vi "NavigateTryingToKeepPath.vi"(1 "Move Type":T1(ring)) -> ()   [LabVIEW 2015, in "Navigation2017.lvlib"]
uses:
  Navigation2017.lvlib
  MovementControl2017.lvlib
  Vector.ctl
  Navigation2017-util.lvlib
  Navigation2017-SubVIs.lvlib
  PathfindingSettings.ctl
  MovementSettings.ctl
  PathCostWeights.ctl
  IntermediatePositionGrids.ctl
panel:
  in  "Reached Next Path Point Threshold Distance (m)":dbl(knob) scale=0.0..1.0
  in  "Time to move 1m (TODO: consider speed?)":u32
  in  "Robot Speed":dbl(slide) scale=0.0..1.0
  in  "Dead Reckoning Move Distance (m)":dbl(knob) scale=0.5..4.0
  in  "Turning Radius (m)":dbl(knob) scale=0.75..4.0
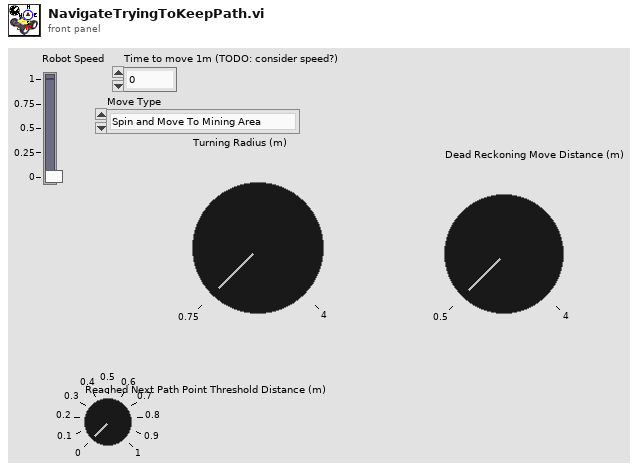
[diagram p1: front panel]
types:
  T1 = enum16{"Spin and Move To Mining Area", "Move To Collector Trough", "Move To Mining Area"}
  T2 = typedef "Navigation2017.lvlib/Vector.ctl" = cluster{"x":dbl, "y":dbl, "angle":dbl}
  T3 = typedef "LocalizationStatus.ctl" = cluster{"x":dbl, "y":dbl, "angle":dbl, "valid":bool, "lastUpdatedTime":dbl}
  T4 = typedef "Navigation2017.lvlib/PathfindingSettings.ctl" = cluster{"Movement Settings":T5, "Dead Zone":dbl, "Max Moves":dbl, "Move Segment Length (m)":dbl, "Path Cost Weights":T6, "Desperation - Reduction Per Attempt (Ratio)":dbl, "Desperation - Max Attempts":i16, "Log All Move Points":bool, "Intermediate Position Grids":T7}
  T5 = typedef "Navigation2017.lvlib/MovementSettings.ctl" = cluster{"Arrival Tolerance (m)":dbl, "Closeness Threshold (m)":dbl, "Pit Obstacle Radius (m)":dbl, "Pit Locations":cluster{"x":dbl, "y":dbl}[]}
  T6 = typedef "Navigation2017.lvlib/PathCostWeights.ctl" = cluster{"Length Weight":dbl, "Angle Weight":dbl, "Angle Error Weight":dbl, "Angle Error Threshold":dbl, "Per Move Penalty":dbl, "Closeness Weight":dbl, "Too Short Penalty":dbl, "Too Short Threshold":dbl}
  T7 = typedef "Navigation2017.lvlib/IntermediatePositionGrids.ctl" = cluster{"x1":dbl, "x2":dbl, "resolution":dbl}[]
  T8 = typedef "Navigation2017.lvlib/PathOfMoves.ctl" = cluster{"Dest Angle Error":dbl, "Dest Angle Considered":bool, "Moves":T9[]}
  T9 = typedef "Navigation2017.lvlib/Move.ctl" = cluster{"Did Reach Dest":bool, "Did Collide":bool, "Sum of Angle Changes (rad)":dbl, "Move Length (m)":dbl, "Closeness Sum":dbl, "Positions Along Move":cluster{"x":dbl, "y":dbl, "angle":dbl}[], "Moved Fwd":bool}
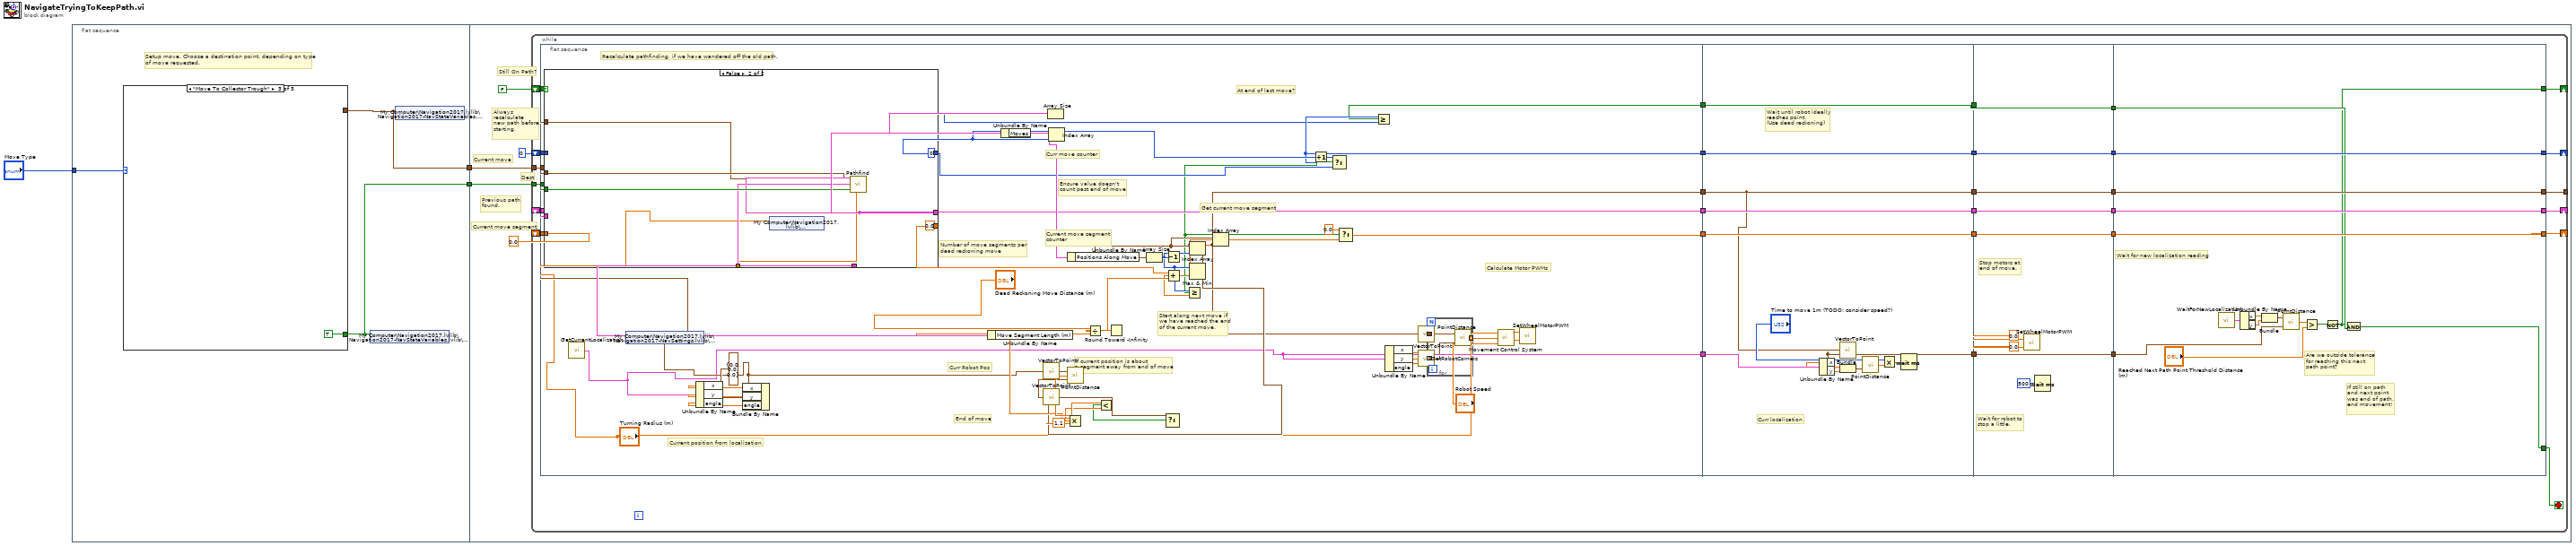
[diagram p0: block diagram]
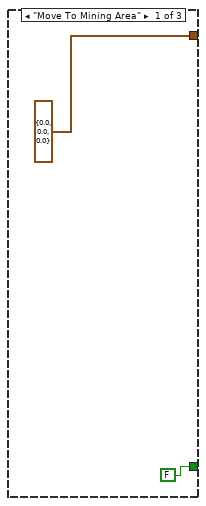
[diagram p2: hidden frame]
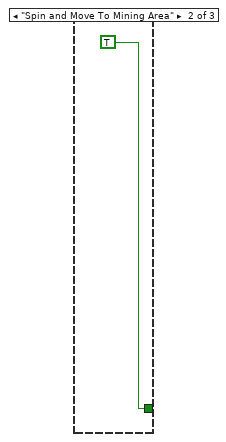
[diagram p3: hidden frame]
diagram:
  n1 = flat-sequence {
    tunnel: "Move Type" -> [w6]
    tunnel: [w5] -> w2
    tunnel: [w4] -> w1
    tunnel: w2 -> [w14]
    tunnel: w1 -> [w13]
    frame #0 {
      # "Setup move. Choose a destination point, depending on type\nof move requested."
      n2 = case shown="\"Move To Collector Trough\"" w6 {
        tunnel: [T2 {"x"=0.0, "y"=0.0, "angle"=0.0} ("Vector") _ _] -> w4
        tunnel: [FALSE TRUE TRUE] -> w5
        frame "Move To Mining Area" {
        }
        frame "Spin and Move To Mining Area" {
        }
        frame "Move To Collector Trough" {
        }
      }
      n3 = shared-variable "My Computer\\Navigation2017.lvlib\\Navigation2017-NavStateVariables.lvlib\\SpecifyingEndAngle"(w5) -> ()  [unwired: 1 in, 1 out]
      n4 = shared-variable "My Computer\\Navigation2017.lvlib\\Navigation2017-NavStateVariables.lvlib\\DestinationPoint"(w4) -> ()  [unwired: 1 in, 1 out]
    }
    frame #1 {
      # "Dest"
      # "Current move"
      # "Current move segment"
      # "Always \nrecalculate\nnew path before\nstarting."
      # "Previous path\nfound."
      # "Still On Path?"
      n5 = while {
        tunnel: w14 -> [w45]
        tunnel: w13 -> [w41]
        shift-right: [w42] -> _
        shift-left: _ -> [w43]
        shift-right: [w39] -> _
        shift-left: 0.0 -> [w40]
        shift-right: [w37] -> _
        shift-left: 0 -> [w38]
        tunnel: [w36] -> _
        shift-right: [w20] -> _
        shift-left: FALSE -> [w44]
        stop <- w16 stop-if-true
        n6 = flat-sequence {
          tunnel: w45 -> [w97]
          tunnel: w44 -> [w93]
          tunnel: w43 -> [w92]
          tunnel: w41 -> [w79]
          tunnel: w40 -> [w70]
          tunnel: w38 -> [w65]
          tunnel: [w91] -> w35
          tunnel: [w66] -> w34
          tunnel: [w61] -> w33
          tunnel: [w56] -> w32
          tunnel: [w46] -> w31
          tunnel: [w47] -> w17
          tunnel: w35 -> [w124]
          tunnel: w34 -> [w123]
          tunnel: w33 -> [w122]
          tunnel: w32 -> [w118]
          tunnel: w31 -> [w116]
          tunnel: [w124] -> w30
          tunnel: [w123] -> w29
          tunnel: [w122] -> w28
          tunnel: [w118] -> w27
          tunnel: [w113] -> w21
          tunnel: [w112] -> w18
          tunnel: w17 -> [w112]
          tunnel: w30 -> [w133]
          tunnel: w29 -> [w132]
          tunnel: w28 -> [w131]
          tunnel: w27 -> [w130]
          tunnel: [w133] -> w26
          tunnel: [w132] -> w25
          tunnel: [w131] -> w24
          tunnel: [w130] -> w23
          tunnel: [w126] -> w22
          tunnel: w21 -> [w126]
          tunnel: [w125] -> w19
          tunnel: w18 -> [w125]
          tunnel: [w145] -> w36
          tunnel: [w146] -> w37
          tunnel: [w147] -> w39
          tunnel: [w148] -> w42
          tunnel: w26 -> [w148]
          tunnel: w25 -> [w147]
          tunnel: w24 -> [w146]
          tunnel: w23 -> [w145]
          tunnel: w22 -> [w143]
          tunnel: [w134] -> w20
          tunnel: w19 -> [w135]
          tunnel: [w137] -> w16
          frame #0 {
            # "Calculate Motor PWMs"
            # "Get current move segment"
            # "At end of last move?"
            # "Curr move counter"
            # "Recalculate pathfinding, if we have wandered off the old path."
            # "Start along next move if\nwe have reached the end\nof the current move."
            # "Ensure value doesn't\ncount past end of move"
            # "Current move segment\ncounter"
            # "Curr Robot Pos"
            # "End of move"
            # "If current position is about \na segment away from end of move"
            # "Current position from localization"
            # "Number of move segments per\ndead reckoning move"
            n7 = call "GetCurrentLocalization.vi"() -> ("Current Localization Status"=w46:T3)
            n8 = shared-variable "My Computer\\Navigation2017.lvlib\\Navigation2017-NavSettings.lvlib\\PathfindingSettings"() -> (w96:T4)  [unwired: 1 in, 1 out]
            n9 = Unbundle By Name(w46) -> ("x"=w83:dbl, "y"=w84:dbl, "angle"=w85:dbl)
            n10 = Bundle By Name(cluster=T2 {"x"=0.0, "y"=0.0, "angle"=0.0} ("Vector"), "x"=w83, "y"=w84, "angle"=w85) -> (w82:T2)
            n11 = case shown="False" w93 {
              tunnel: w97 -> [_ w111]
              tunnel: w96 -> [_ w110]
              tunnel: [w103 w109] -> w91
              tunnel: w79 -> [_ w108]
              tunnel: w92 -> [w103 _]
              tunnel: w82 -> [_ w107]
              tunnel: w70 -> [w102 _]
              tunnel: [w102 0.0] -> w69
              tunnel: w65 -> [w101 _]
              tunnel: [w101 0] -> w63
              tunnel: "Turning Radius (m)" -> [_ w104]
              frame True {
              }
              frame False {
                n12 = shared-variable "My Computer\\Navigation2017.lvlib\\Navigation2017-NavSettings.lvlib\\TurnRadius"(w104) -> ()  [unwired: 1 in, 1 out]
                n13 = call "Pathfind.vi"("Start Vector"=w107, "Destination"=w108, "Pathfinding Settings"=w110, "Specified End Angle"=w111, "Turn Radius (m)"=w104) -> ("Best Path"=w109:T8)  [unwired: 3 out]
              }
            }
            n14 = Unbundle By Name(w96) -> ("Move Segment Length (m)"=w88:dbl)
            n15 = Unbundle By Name(w91) -> ("Moves"=w60:T9[])
            n16 = call "VectorToPoint.vi"("Vector"=w82) -> ("Point"=w81:cluster{"x":dbl, "y":dbl})
            n17 = Array Size(array=w60) -> (size(s)=w59:i32)
            n18 = Index Array(array=w60, index=w63) -> (element=w94:T9)
            n19 = Unbundle By Name(w94) -> ("Positions Along Move"=w73:cluster{"x":dbl, "y":dbl, "angle":dbl}[])
            n20 = Multiply(x=w88, y=1.1) -> (x*y=w87:dbl)
            n21 = Divide(x="Dead Reckoning Move Distance (m)", y=w88) -> (x/y=w77:dbl)
            n22 = Round Toward -Infinity(1:w77) -> (0:w74:dbl)
            n23 = Array Size(array=w73) -> (size(s)=w76:i32)
            n24 = Decrement(x=w76) -> (x-1=w71:i32)
            n25 = Add(x=w69, y=w74) -> (x+y=w72:dbl)
            n26 = Greater Or Equal?(x=w71, y=w72) -> (x >= y?=w62:bool)
            n27 = Index Array(array=w73, index=w71) -> (element=w75:cluster{"x":dbl, "y":dbl, "angle":dbl})
            n28 = call "VectorToPoint.vi"("Vector"=w75) -> ("Point"=w78:cluster{"x":dbl, "y":dbl})
            n29 = call "PointDistance.vi"("Point 2"=w78, "Point 1"=w81) -> ("Distance"=w90:dbl)
            n30 = Less?(x=w90, y=w87) -> (x < y?=w80:bool)
            n31 = Select(t=w78, s=w80) -> ()  [unwired: 1 in, 1 out]
            n32 = Max & Min(x=w71, y=w72) -> (min(x,y)=w68:dbl)  [unwired: 1 out]
            n33 = Index Array(array=w73, index=w68) -> (element=w56:cluster{"x":dbl, "y":dbl, "angle":dbl})
            n34 = Increment(x=w63) -> (x+1=w64:i32)
            n35 = Select(t=w64, s=w62, f=w63) -> (s? t:f=w61:i32)
            n36 = Select(t=0.0, s=w62, f=w68) -> (s? t:f=w66:dbl)
            n37 = Greater Or Equal?(x=w61, y=w59) -> (x >= y?=w47:bool)
            n38 = Unbundle By Name(w46) -> ("x"=w52:dbl, "y"=w51:dbl, "angle"=w50:dbl)
            n39 = call "VectorToPoint.vi"("Vector"=w56) -> ("Point"=w55:cluster{"x":dbl, "y":dbl})
            n40 = call "GetRobotCorners.vi"("botAngle (rad)"=w50, "botY (m)"=w51, "botX (m)"=w52) -> ("Corner Points (m)"=w58:cluster{dbl, dbl}[])
            n41 = for {
              tunnel: w58 -> [w99] mode=indexing
              tunnel: [w98] -> w57 mode=indexing
              tunnel: w55 -> [w100]
              n42 = call "PointDistance.vi"("Point 2"=w99, "Point 1"=w100) -> ("Distance"=w98:dbl)
            }
            n43 = call "Movement Control System.vi"("Turning Radius"="Turning Radius (m)", "Corner Distances"=w57, "Speed"="Robot Speed") -> ("Left Side PWM"=w49:dbl, "Right Side PWM"=w48:dbl)  [unwired: 4 out]
            n44 = call "SetWheelMotorPWM.vi"("Right Motor PWM"=w48, "Left Motor PWM"=w49) -> ()
          }
          frame #1 {
            # "Wait until robot ideally\nreaches point.\n(Use dead reckoning)"
            # "Curr localization"
            n45 = Unbundle By Name(w116) -> ("x"=w115:dbl, "y"=w114:dbl)
            n46 = call "VectorToPoint.vi"("Vector"=w118) -> ("Point"=w113:cluster{"x":dbl, "y":dbl})
            n47 = Bundle("x"=w115, "y"=w114) -> (w117:cluster{"x":dbl, "y":dbl})  [unwired: 1 in]
            n48 = call "PointDistance.vi"("Point 2"=w117, "Point 1"=w113) -> ("Distance"=w120:dbl)
            n49 = Multiply(x="Time to move 1m (TODO: consider speed?)", y=w120) -> (x*y=w119:dbl)
            n50 = Wait (ms)(milliseconds to wait=w119) -> ()  [unwired: 1 out]
          }
          frame #2 {
            # "Wait for robot to\nstop a little."
            # "Stop motors at\nend of move."
            n51 = call "SetWheelMotorPWM.vi"("Right Motor PWM"=0.0 ("Right Motor Speed"), "Left Motor PWM"=0.0 ("Left Motor Speed")) -> ()
            n52 = Wait (ms)(milliseconds to wait=u32 500) -> ()  [unwired: 1 out]
          }
          frame #3 {
            # "If still on path\nand next point\nwas end of path,\nend movement!"
            # "Are we outside tolerance\nfor reaching this next\npath point?"
            # "Wait for new localization reading"
            n53 = call "WaitForNewLocalization.vi"() -> ("Localization Status"=w144:T3)
            n54 = Unbundle By Name(w144) -> ("x"=w142:dbl, "y"=w141:dbl)
            n55 = Bundle("x"=w142, "y"=w141) -> (w140:cluster{"x":dbl, "y":dbl})  [unwired: 1 in]
            n56 = call "PointDistance.vi"("Point 2"=w143, "Point 1"=w140) -> ("Distance"=w139:dbl)
            n57 = Greater?(x=w139, y="Reached Next Path Point Threshold Distance (m)") -> (0:w136:bool)
            n58 = Not(x=w136) -> (.not. x?=w134:bool)
            n59 = And(x=w134, y=w135) -> (x .and. y?=w137:bool)
          }
        }
      }
    }
  }
